vi "Fix BDPW Checksum.vi"(9 "Terminal Counts":T1, 10 "Only fix 3rd hash (F)":bool, 11 "Resources in":T2) -> (3 "Resources out":T2)   [LabVIEW 2015]
uses:
  Resource Array.ctl
  Resource.ctl
  <userlib>/_OpenG.lib/md5/md5.llb/MD5 Message Digest (Binary String)__ogtk.vi
  Find Resource by Type (String).vi
panel:
  # "Thank you Thomas Zeugner! You saved me the trouble of figuring out how this checksum works. :)\nAdapted from https://github.com/tomsoftware/VI-Explorer/blob/master/php/clBDPW.php"
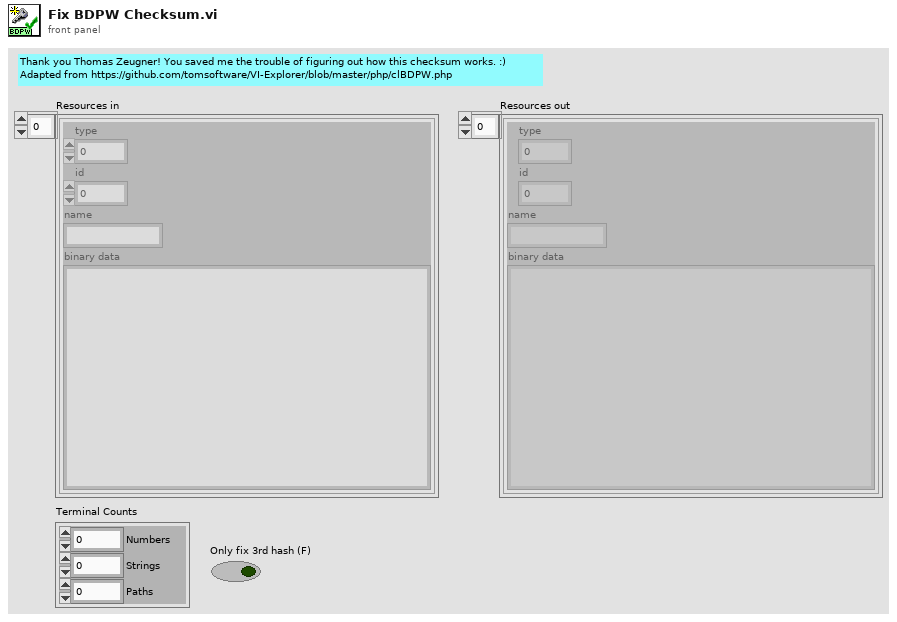
[diagram p1: front panel]
types:
  T1 = cluster{"Numbers":u32, "Strings":u32, "Paths":u32}
  T2 = typedef "Resource Array.ctl" = T3[]
  T3 = typedef "Resource.ctl" = cluster{"type":u32, "id":i32, "name":string, "binary data":string}
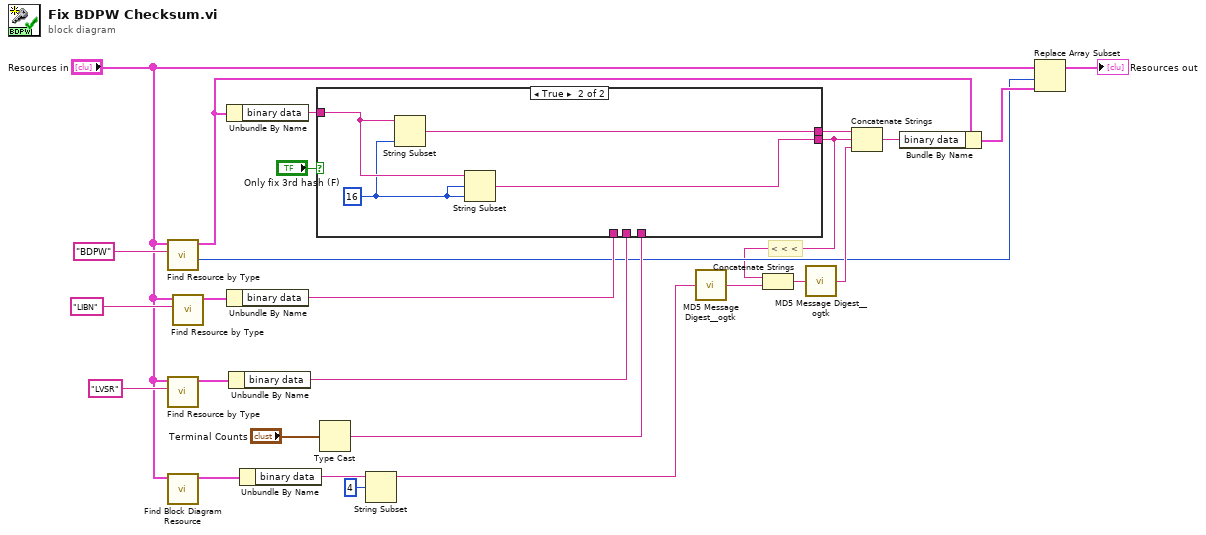
[diagram p0: block diagram]
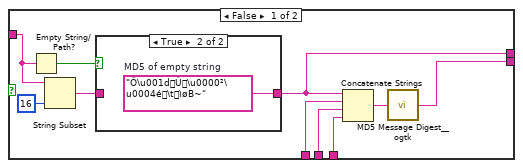
[diagram p2: hidden frame]
diagram:
  # "< < <"
  n1 = call-poly "Find Resource by Type.vi"("Resource Type"="BDPW", "Resources"="Resources in") -> ("Index"=w10:i32, "Resource"=w9:T3)  [unwired: 7 in, 1 out]
  n2 = call-poly "Find Resource by Type.vi"("Resource Type"="LVSR", "Resources"="Resources in") -> ("Resource"=w24:T3)  [unwired: 7 in, 2 out]
  n3 = call "Find Block Diagram Resource.vi"("Resources"="Resources in") -> ("Resource"=w6:T3)  [unwired: 8 in, 2 out]
  n4 = call-poly "Find Resource by Type.vi"("Resource Type"="LIBN", "Resources"="Resources in") -> ("Resource"=w25:T3)  [unwired: 7 in, 2 out]
  n5 = Unbundle By Name(w9) -> ("binary data"=w3:string)
  n6 = Unbundle By Name(w25) -> ("binary data"=w23:string)
  n7 = Unbundle By Name(w24) -> ("binary data"=w22:string)
  n8 = Unbundle By Name(w6) -> ("binary data"=w14:string)
  n9 = Type Cast(x="Terminal Counts") -> (*(type *) &x=w20:string)  [unwired: 1 in]
  n10 = case shown="True" "Only fix 3rd hash (F)" {
    tunnel: w23 -> [w35 _]
    tunnel: w22 -> [w34 _]
    tunnel: w20 -> [w32 _]
    tunnel: [w31 w39] -> w2
    tunnel: [w30 w40] -> w4
    tunnel: w3 -> [w28 w42]
    frame False {
      n11 = Empty String/Path?(string/path=w28) -> (empty?=w27:bool)
      n12 = String Subset(string=w28, length (rest)=16 ("length (rest)")) -> (substring=w29:string)  [unwired: 1 in]
      n13 = case shown="True" w27 {
        tunnel: [w37 w38] -> w30
        tunnel: w29 -> [w37 _]
        frame False {
        }
        frame True {
          w38 = "Ô\u001dÙ\u0000²\u0004é\tìøB~"  # MD5 of empty string
        }
      }
      n14 = Concatenate Strings(w30, w35, w34, w32) -> (w33:string)
      n15 = call-poly <userlib>:"MD5 Message Digest__ogtk.vi"("Message"=w33) -> ("MD5 Message Digest"=w31:string)
    }
    frame True {
      w41 = 16 ("length (rest)")
      n16 = String Subset(string=w42, length (rest)=w41) -> (substring=w40:string)  [unwired: 1 in]
      n17 = String Subset(string=w42, offset (0)=w41, length (rest)=w41) -> (substring=w39:string)
    }
  }
  n18 = String Subset(string=w14, offset (0)=4) -> (substring=w12:string)  [unwired: 1 in]
  n19 = call-poly <userlib>:"MD5 Message Digest__ogtk.vi"("Message"=w12) -> ("MD5 Message Digest"=w13:string)
  n20 = Concatenate Strings(w2, w13) -> (w16:string)
  n21 = call-poly <userlib>:"MD5 Message Digest__ogtk.vi"("Message"=w16) -> ("MD5 Message Digest"=w15:string)
  n22 = Concatenate Strings(w4, w2, w15) -> (w19:string)
  n23 = Bundle By Name(cluster=w9, "binary data"=w19) -> (w18:T3)
  n24 = Replace Array Subset(array="Resources in", new element=w18, index=w10) -> (→"Resources out":T2)
